vi "ai_oneshot_lite.vi"() -> ()   [LabVIEW 2020]
uses:
  <vilib>/Analysis/baseanly.llb/Mean (DBL).vi
  <vilib>/Analysis/NI_AALBase.lvlib
panel:
  out "数组":dbl[](array[numeric]) format="%_6g"
  in  "AiOneShotPoints":u32=1000
  out "error out":errorcluster caption="错误输出"
  out "AiFifoResidual":i32
  out "波形图":sgl[][](graph)
  in  "SamplePeriod(ns)":u32=5000
  in  "ChanSel":bool[](array[boolean])=[TRUE, TRUE, TRUE, TRUE, TRUE, TRUE, TRUE, TRUE, FALSE, FALSE, FALSE, FALSE, FALSE, FALSE, FALSE, FALSE, FALSE, FALSE, FALSE, FALSE, FALSE, FALSE, FALSE, FALSE]
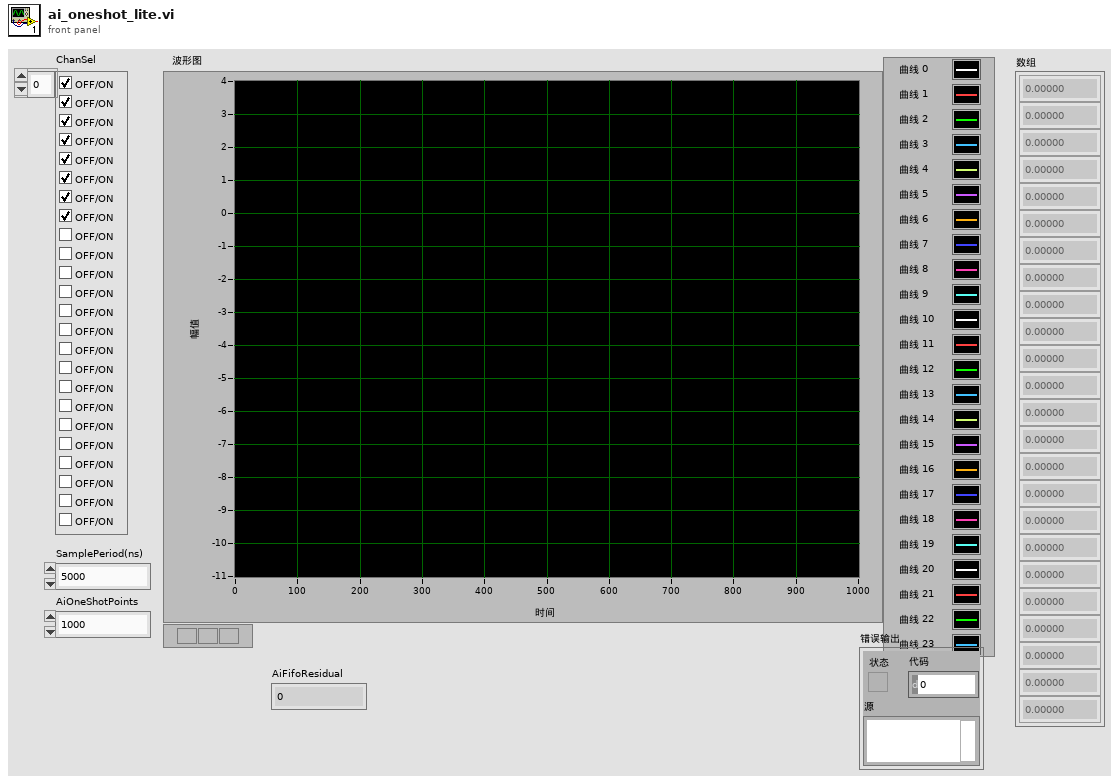
[diagram p1: front panel]
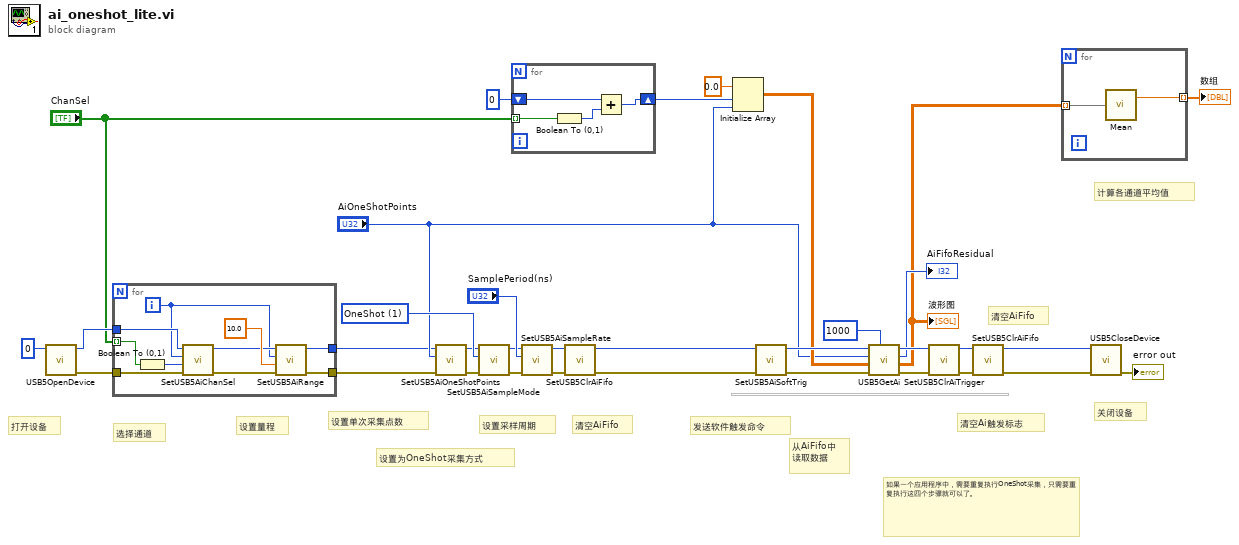
[diagram p0: block diagram]
diagram:
  w30 = u8 1 items=["Continuous", "OneShot"] ("AiSampleMode")
  # "设置量程"
  # "计算各通道平均值"
  # "关闭设备"
  # "如果一个应用程序中，需要重复执行OneShot采集，只需要重复执行这四个步骤就可以了。"
  # "清空AiFifo"
  # "清空Ai触发标志"
  # "从AiFifo中\n读取数据"
  # "发送软件触发命令"
  # "清空AiFifo"
  # "设置采样周期"
  # "设置为OneShot采集方式"
  # "设置单次采集点数"
  # "选择通道"
  # "打开设备"
  n1 = call "USB5OpenDevice.vi"("DevIndex"=0) -> ("error out"=w32:errorcluster, "DevIndex Out"=w33:i32)  [unwired: 9 in]
  n2 = for {
    tunnel: w33 -> [w44]
    tunnel: w32 -> [w43]
    tunnel: [w36] -> w4
    tunnel: [w35] -> w3
    tunnel: "ChanSel" -> [w41] mode=indexing
    i -> [w37]
    n3 = Boolean To (0,1)(Boolean=w41) -> (0, 1=w42:i16)
    n4 = call "SetUSB5AiChanSel.vi"("错误输入（无错误）"=w43, "Sel"=w42, "Chan"=w37, "DevIndex"=w44) -> ("错误输出"=w38:errorcluster, "DevIndex Out"=w39:i32)  [unwired: 6 in]
    n5 = call "SetUSB5AiRange.vi"("错误输入（无错误）"=w38, "AiRange"=sgl 10.0, "Chan"=w37, "DevIndex"=w39) -> ("错误输出"=w35:errorcluster, "DevIndex Out"=w36:i32)  [unwired: 6 in]
  }
  n6 = call "SetUSB5AiOneShotPoints.vi"("错误输入（无错误）"=w3, "AiOneShotPoints"="AiOneShotPoints", "DevIndex"=w4) -> ("错误输出"=w11:errorcluster, "DevIndex Out"=w12:i32)  [unwired: 7 in]
  n7 = call "SetUSB5AiSampleMode.vi"("错误输入（无错误）"=w11, "AiSampleMode"=w30, "DevIndex"=w12) -> ("错误输出"=w16:errorcluster, "DevIndex Out"=w17:i32)  [unwired: 7 in]
  n8 = for {
    tunnel: "ChanSel" -> [w48] mode=indexing
    shift-right: [w45] -> w18
    shift-left: i16 0 -> [w46]
    n9 = Boolean To (0,1)(Boolean=w48) -> (0, 1=w47:i16)
    n10 = Add(x=w46, y=w47) -> (x+y=w45:i16)
  }
  n11 = call "SetUSB5AiSampleRate.vi"("错误输入（无错误）"=w16, "SamplePeriod(ns)"="SamplePeriod(ns)", "DevIndex"=w17) -> ("错误输出"=w14:errorcluster, "DevIndex Out"=w15:i32)  [unwired: 7 in]
  n12 = call "SetUSB5ClrAiFifo.vi"("错误输入（无错误）"=w14, "DevIndex"=w15) -> ("错误输出"=w28:errorcluster, "DevIndex Out"=w29:i32)  [unwired: 8 in]
  n13 = Initialize Array(sgl 0.0 ("元素"), w18, "AiOneShotPoints") -> (w22:sgl[][])
  n14 = call "SetUSB5AiSoftTrig.vi"("错误输入（无错误）"=w28, "DevIndex"=w29) -> ("错误输出"=w26:errorcluster, "DevIndex Out"=w27:i32)  [unwired: 8 in]
  n15 = call "USB5GetAi.vi"("TimeOut"=1000, "错误输入（无错误）"=w26, "Ai"=w22, "Points"="AiOneShotPoints", "DevIndex"=w27) -> ("错误输出"=w7:errorcluster, "Ai Out"=w1:sgl[][], "AiFifoUsed"=→"AiFifoResidual":i32, "DevIndex Out"=w8:i32)  [unwired: 3 in]
  "波形图" <- w1
  n16 = call "SetUSB5ClrAiTrigger.vi"("错误输入（无错误）"=w7, "DevIndex"=w8) -> ("错误输出"=w6:errorcluster, "DevIndex Out"=w9:i32)  [unwired: 8 in]
  n17 = call "SetUSB5ClrAiFifo.vi"("错误输入（无错误）"=w6, "DevIndex"=w9) -> ("错误输出"=w21:errorcluster, "DevIndex Out"=w20:i32)  [unwired: 8 in]
  n18 = for {
    tunnel: w1 -> [w50] mode=indexing
    tunnel: [w49] -> w2 mode=indexing
    n19 = call-poly <vilib>:"Mean.vi"("X"=w50) -> ("mean"=w49:dbl)  [unwired: 1 out]
  }
  "数组" <- w2
  n20 = call "USB5CloseDevice.vi"("错误输入（无错误）"=w21, "DevIndex"=w20) -> ("error out"=→"error out":errorcluster)  [unwired: 8 in, 1 out]
